vi "dsdll_output_write_byte_array.vi"(5 "volume (1: don't change volume)":i32=1 min=-10000 max=1 step=1, 7 "play (true)":bool=TRUE, 8 "error in":errorcluster, 9 "looped mode (true)":bool=TRUE, 10 "byte data":u8[](array[numeric]), 11 "dsdll instance in":T1={"dsdll path"=path "E:/LVprog/DirectSoundDLL/dsdll.dll", "dsdll handle"=[], "output devices"=[], "capture devices"=[]}) -> (0 "error out":errorcluster, 3 "dsdll instance out":T1)   [LabVIEW 2013, in "dsdll.lvlib"]
doc: "Call this to write raw sample data into the output device buffer. \nOptionally starts playback and sets volume. If the 'volume' input left unconnectged it does not change the volume. The range of the volume is {-10000 to 0} where -10000 is equal to -100dB and 0 is 0dB (full volume).\nThe 'looped mode' option enables playback of the waveform in an infinite loop. If set to false the waveform will be played just once.\n\nData are expected in little-endian channel interleaved format. Example for PCM 16 bit, 2 channels (s - sample, c - channel, b0/b1 - low/high sample byte):\n[s0c0b0, s0c0b1, s0c1b0, s0c1b1, s1c0b0, s1c0b1, s1c1b0, s1c1b1, ...]"
uses:
  dsdll.lvlib
  dsdll_instance.ctl
  dsdll_device_record.ctl
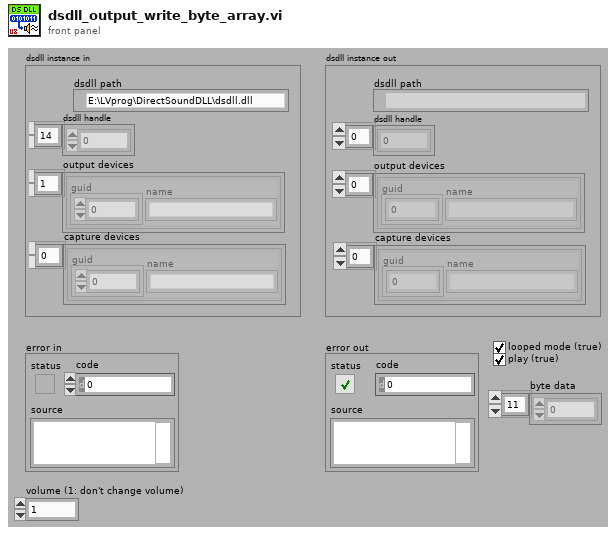
[diagram p1: front panel]
types:
  T1 = typedef "dsdll.lvlib/dsdll_instance.ctl" = cluster{"dsdll path":path, "dsdll handle":u8[], "output devices":T2[], "capture devices":T2[]}
  T2 = typedef "dsdll.lvlib/dsdll_device_record.ctl" = cluster{"guid":u8[], "name":string}
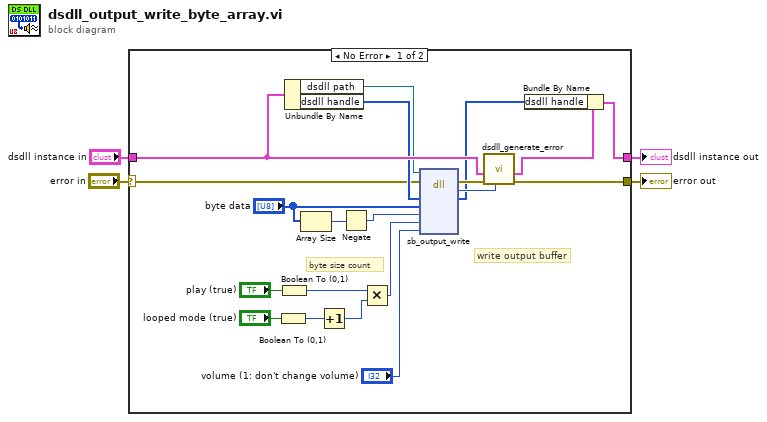
[diagram p0: block diagram]
diagram:
  n1 = case shown="No Error" "error in" {
    selector: "error in" -> [w15 w25]
    tunnel: "dsdll instance in" -> [w22 w26]
    tunnel: [w19 w25] -> w3
    tunnel: [w16 w26] -> w4
    frame No Error {
      # "byte size count"
      # "write output buffer"
      n2 = Boolean To (0,1)(Boolean="looped mode (true)") -> (0, 1=w7:i16)
      n3 = Boolean To (0,1)(Boolean="play (true)") -> (0, 1=w8:i16)
      n4 = Unbundle By Name(w22) -> ("dsdll path"=w21:path, "dsdll handle"=w20:u8[])
      n5 = Array Size(array="byte data") -> (size(s)=w12:i32)
      n6 = Increment(x=w7) -> (x+1=w5:i16)
      n7 = Negate(x=w12) -> (-x=w11:i32)
      n8 = Multiply(x=w8, y=w5) -> (x*y=w6:i16)
      n9 = dll-call lib="dsdll.dll" fn="sb_output_write" ("sb_get_handle_size()")(path in=w21, error in=w15, "handle"=w20, "data"="byte data", "count"=w11, "play"=w6, "volume"="volume (1: don't change volume)") -> (error out=w24:errorcluster, "error"=w23:i32, "handle"=w17:u8[])  [unwired: 5 in, 1 out]
      n10 = call "dsdll_generate_error.vi"("error code"=w23, "error in"=w24, "dsdll instance in"=w22) -> ("error out"=w19:errorcluster, "dsdll instance out"=w18:T1)  [unwired: 6 in, 1 out]
      n11 = Bundle By Name(cluster=w18, "dsdll handle"=w17) -> (w16:T1)
    }
    frame Error {
    }
  }
  "error out" <- w3
  "dsdll instance out" <- w4
